vi "Alp Dev Control Ex.vi"(8 "error in (no error)":errorcluster, 9 "UserStructPtr":u32, 10 "ControlType":i32, 11 "DeviceId":u32) -> (0 "error out":errorcluster, 1 "UserStructPtr out":u32, 3 "function return":i32)   [LabVIEW 2013, in "alpD41.lvlib"]
uses:
  <userlib>/alpD41/alpD41.lvlib
  <userlib>/alpD41/alpD41.dll
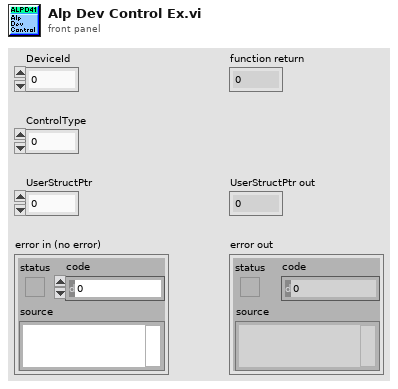
[diagram p1: front panel]
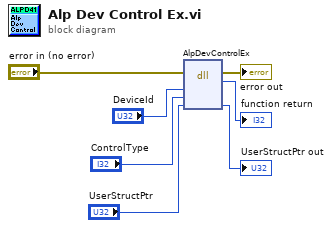
[diagram p0: block diagram]
diagram:
  n1 = dll-call lib="C:/Program Files (x86)/National Instruments/LabVIEW 2013/user.lib/alpD41/alpD41.*" fn="AlpDevControlEx"(error in="error in (no error)", "DeviceId"="DeviceId", "ControlType"="ControlType", "UserStructPtr"="UserStructPtr") -> (error out=→"error out":errorcluster, →"function return":i32, "UserStructPtr"=→"UserStructPtr out":u32)  [unwired: 4 in, 1 out]
